vi "Ej 12 NododePropiedad.vi"() -> ()   [LabVIEW 2021]
panel:
  out "Waveform Chart":dbl(graph)
  in  "Posicion horizontal":dbl(slide) scale=0.0..400.0
  out "Cadena caracteres":string
  in  "Posicion vertical":dbl(slide) scale=0.0..300.0
  in  "Deshabilitar":bool
  in  "Boolean":bool
  in  "Limite":dbl
  in  "stop":bool
  out "Tank":dbl(slide) scale=0.0..10.0
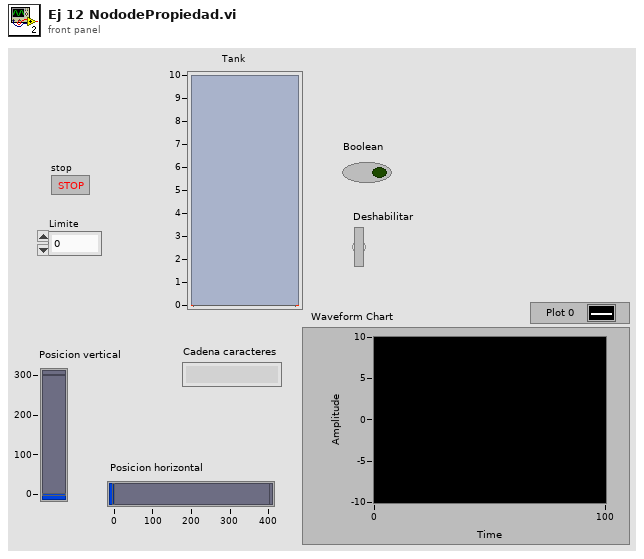
[diagram p1: front panel]
types:
  T1 = cluster{"Posicion horizontal":dbl, "Posicion vertical":dbl}
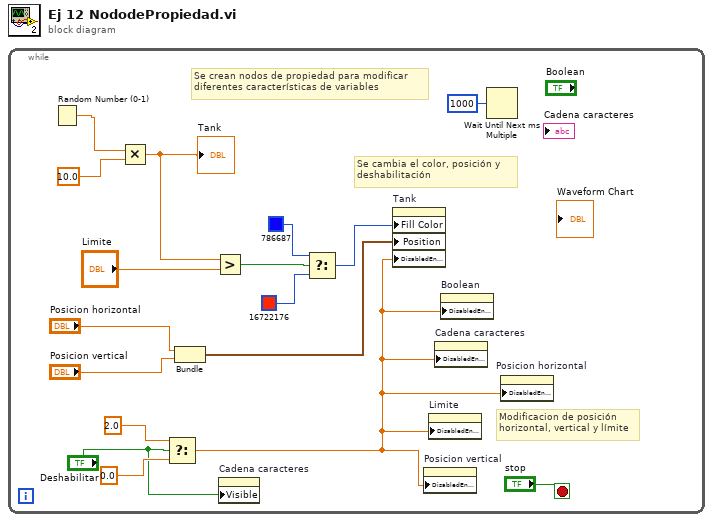
[diagram p0: block diagram]
diagram:
  n1 = while {
    stop <- "stop" stop-if-true
    # "Se cambia el color, posición y \ndeshabilitación"
    # "Modificacion de posición \nhorizontal, vertical y límite"
    # "Se crean nodos de propiedad para modificar\ndiferentes características de variables"
    n2 = Random Number (0-1)() -> (number: 0 to 1=w16:dbl)
    n3 = Multiply(x=w16, y=10.0) -> (x*y=w13:dbl)
    "Tank" <- w13
    n4 = Select(t=2.0, s="Deshabilitar", f=0.0) -> (s? t:f=w2:dbl)
    n5 = Bundle("Posicion horizontal"="Posicion horizontal", "Posicion vertical"="Posicion vertical") -> (w3:T1)  [unwired: 1 in]
    n6 = Greater?(x=w13, y="Limite") -> (0:w12:bool)
    n7 = property on="Cadena caracteres" class="Str"("Visible"="Deshabilitar") -> ()  [unwired: 2 in, 2 out]
    n8 = Select(t=u32 786687, s=w12, f=u32 16722176) -> (s? t:f=w8:u32)
    n9 = property on="Tank" class="Slide (strict)"("Fill Color"=w8, "Position"=w3, "DisabledEnum"=w2) -> ()  [unwired: 2 in, 2 out]
    n10 = property on="Posicion vertical" class="Slide (strict)"("DisabledEnum"=w2) -> ()  [unwired: 2 in, 2 out]
    n11 = property on="Limite" class="DigNum (strict)"("DisabledEnum"=w2) -> ()  [unwired: 2 in, 2 out]
    n12 = property on="Cadena caracteres" class="Str"("DisabledEnum"=w2) -> ()  [unwired: 2 in, 2 out]
    n13 = property on="Boolean" class="Bool (strict)"("DisabledEnum"=w2) -> ()  [unwired: 2 in, 2 out]
    n14 = Wait Until Next ms Multiple(millisecond multiple=u32 1000) -> ()  [unwired: 1 out]
    n15 = property on="Posicion horizontal" class="Slide (strict)"("DisabledEnum"=w2) -> ()  [unwired: 2 in, 2 out]
  }
